vi "test Correct Scheduled Labels In Log.vi"(8 "error in":errorcluster, 11 "TestCase in":refnum<class "Logging Loopback.lvclass">) -> (0 "error out":errorcluster, 3 "TestCase out":refnum<class "Logging Loopback.lvclass">)   [LabVIEW 2020, in "Logging Loopback.lvclass"]
uses:
  Logging Loopback.lvclass
  Logging Loopback.lvclass/Logging Loopback.ctl
  6070ecc1-7a7f-4aba-84f3-8f274e3c644e.vi
  <vilib>/WebDAVClient/Advanced/Get Buffer.vi
  <vilib>/addons/_JKI Toolkits/VI Tester/TestCase.llb/TestCase.lvclass
  <vilib>/WebDAVClient/NI_WebDAV.lvlib
  C:/Program Files (x86)/National Instruments/LabVIEW 2020/vi.lib/addons/_JKI Toolkits/VI Tester/TestCase.llb/TestCase.lvclass
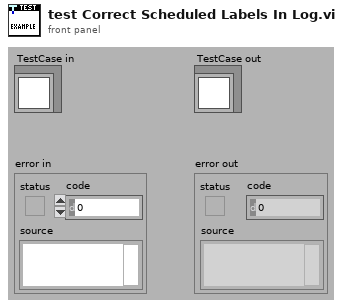
[diagram p1: front panel]
types:
  T1 = typedef "NI_WebDAV.lvlib/SessionHandle.ctl" = refnum<k1>
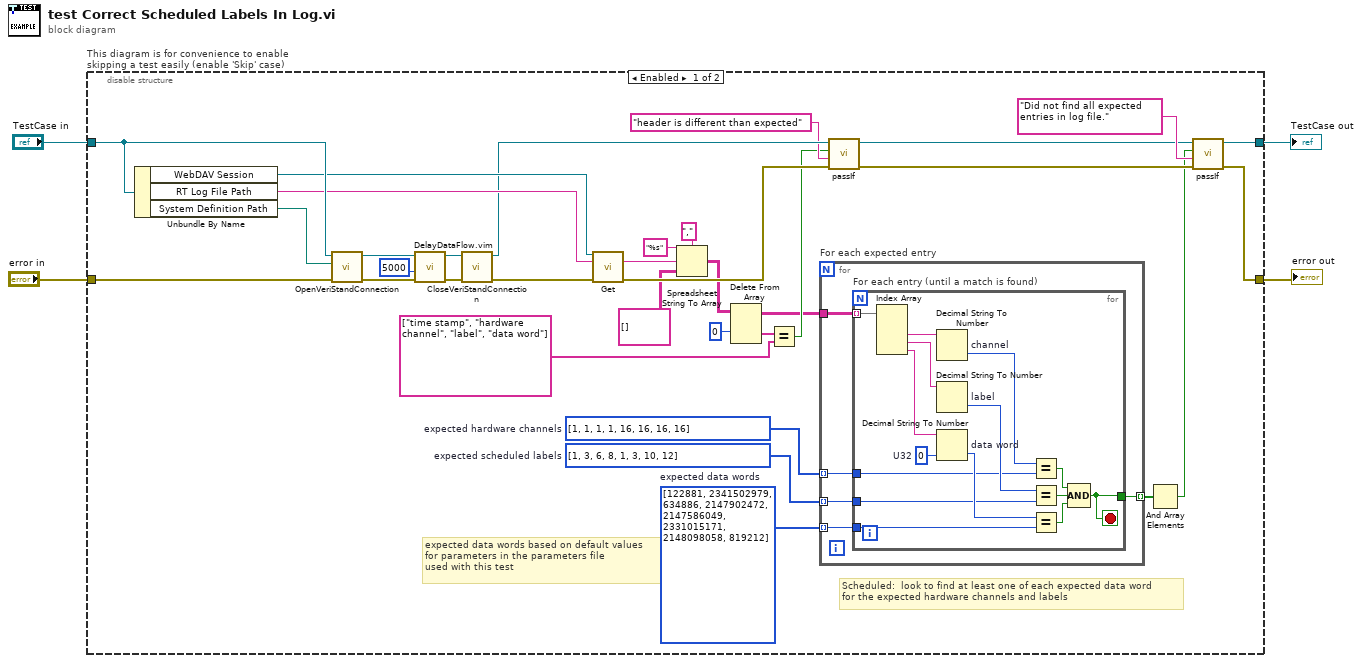
[diagram p0: block diagram]
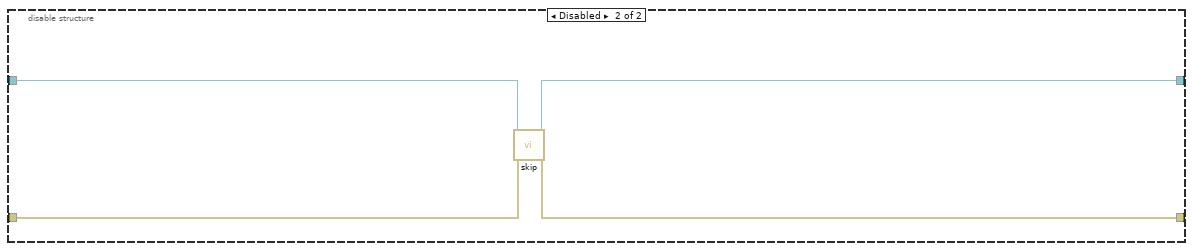
[diagram p2: hidden frame]
diagram:
  n1 = disable-structure "This diagram is for convenience to enable skipping a test easily (enable 'Skip' case)" shown="Enabled" {
    disable-tunnel: "TestCase in" -> [w34 w61]
    disable-tunnel: [w21 w59] -> w1
    disable-tunnel: [w22 w60] -> w3
    disable-tunnel: "error in" -> [w37 w58]
    frame Enabled {
      w8 = u32[] [122881, 2341502979, 634886, 2147902472, 2147586049, 2331015171, 2148098058, 819212]  # expected data words
      w10 = i32[] [1, 1, 1, 1, 16, 16, 16, 16]  # expected hardware channels
      w9 = i32[] [1, 3, 6, 8, 1, 3, 10, 12]  # expected scheduled labels
      # "Scheduled:  look to find at least one of each expected data word\nfor the expected hardware channels and labels"
      # "expected data words based on default values\nfor parameters in the parameters file\nused with this test"
      n2 = Unbundle By Name(w34) -> ("WebDAV Session"=w28:T1, "RT Log File Path"=w27:string, "System Definition Path"=w35:path)
      n3 = call-dynamic "OpenVeriStandConnection.vi"("error in (no error)"=w37, "System Definition File"=w35, "VeriStand Test Case in"=w34) -> ("error out"=w36:errorcluster, "VeriStand Test Case out"=w31:refnum<class "Logging Loopback.lvclass">)  [unwired: 6 in, 1 out]
      n4 = call "DelayDataFlow.vim"("value in"=w36, "milliseconds to wait"=u32 5000) -> ("value out"=w33:errorcluster)  [unwired: 2 in, 1 out]
      n5 = call-dynamic "CloseVeriStandConnection.vi"("error in (no error)"=w33, "VeriStand Test Case in"=w31) -> ("error out"=w30:errorcluster, "VeriStand Test Case out"=w18:refnum<class "Logging Loopback.lvclass">)  [unwired: 8 in]
      n6 = call-poly <vilib>:"Get.vi"("session handle"=w28, "relative uri"=w27, "error in (no error)"=w30) -> ("data"=w26:string, "error out"=w29:errorcluster)  [unwired: 10 in, 1 out]
      n7 = Spreadsheet String To Array(delimiter (Tab)=",", format string="%s", spreadsheet string=w26, array type (2D Dbl)=string[][] []) -> (array=w15:string[][])
      n8 = Delete From Array(array=w15, index (row)=0) -> (deleted portion=w14:string[], array with subset deleted=w7:string[][])  [unwired: 2 in]
      n9 = Equal?(x=w14, y=string[] ["time stamp", "hardware channel", "label", "data word"]) -> (x = y?=w11:bool)
      n10 = for "For each expected entry" {
        tunnel: w10 -> [w41] mode=indexing
        tunnel: w9 -> [w40] mode=indexing
        tunnel: w8 -> [w39] mode=indexing
        tunnel: w7 -> [w42]
        tunnel: [w38] -> w6 mode=indexing
        n11 = for "For each entry (until a match is found)" {
          tunnel: w42 -> [w57] mode=indexing
          tunnel: w41 -> [w49]
          tunnel: w40 -> [w51]
          tunnel: w39 -> [w53]
          tunnel: [w46] -> w38
          stop <- w46 stop-if-true
          w45 = u32 0  # U32
          n12 = Index Array(array=w57) -> (element #2=w56:string, element #3=w55:string, element #4=w54:string)  [unwired: 4 in, 1 out]
          n13 = Decimal String To Number "channel"(string=w56) -> (number=w48:i32)  [unwired: 2 in, 1 out]
          n14 = Decimal String To Number "label"(string=w55) -> (number=w50:i32)  [unwired: 2 in, 1 out]
          n15 = Decimal String To Number "data word"(string=w54, default (0L)=w45) -> (number=w52:u32)  [unwired: 1 in, 1 out]
          n16 = Equal?(x=w48, y=w49) -> (x = y?=w43:bool)
          n17 = Equal?(x=w50, y=w51) -> (x = y?=w44:bool)
          n18 = Equal?(x=w52, y=w53) -> (x = y?=w47:bool)
          n19 = Compound Arithmetic op=AND(w43, w44, w47) -> (w46:bool)
        }
      }
      n20 = call-dynamic "passIf.vi"("error in (no error)"=w29, "message (\"\")"="header is different than expected" ("message (\"\")"), "pass"=w11, "TestCase in"=w18) -> ("error out"=w19:errorcluster, "TestCase out"=w17:refnum<class "Logging Loopback.lvclass">)  [unwired: 6 in]
      n21 = And Array Elements(Boolean array=w6) -> (logical AND=w5:bool)
      n22 = call-dynamic "passIf.vi"("error in (no error)"=w19, "message (\"\")"="Did not find all expected entries in log file." ("message (\"\")"), "pass"=w5, "TestCase in"=w17) -> ("error out"=w22:errorcluster, "TestCase out"=w21:refnum<class "Logging Loopback.lvclass">)  [unwired: 6 in]
    }
    frame Disabled {
      # "skip test result while test is under development"
      n23 = call <vilib>:"skip.vi"("error in (no error)"=w58, "TestCase in"=w61) -> ("error out"=w60:errorcluster, "TestCase out"=w59:refnum<class "Logging Loopback.lvclass">)  [unwired: 8 in]
    }
  }
  "error out" <- w3
  "TestCase out" <- w1
